vi "SEK2020v1SubVIAlinhar.vi"(9 "Min EV3 Cor":sgl, 10 "Max EV3 Cor":sgl, 11 "NXT/EV3":T1) -> (3 "NXT/EV3 2":T1)   [LabVIEW 2016]
uses:
  <vilib>/NXT/Subs/LVHSConnector.ctl
  <vilib>/NXT/LegoClasses/BrickReference/BrickReference.lvclass
  <vilib>/NXT/Block Support/NXT_OutputPort.ctl
  <vilib>/NXT/Block Support/NXT_InputPort.ctl
  <vilib>/NXT/Dual Mode Library/Sensors/EV3_Color_Reflect.vi
  <vilib>/NXT/NXTIO Xnodes/NXTIONodeSubVIs/NXTMoveMotors.vi
  <vilib>/NXT/NXTIO Xnodes/NXTIONodeSubVIs/NXTStopMotors.vi
  <vilib>/NXT/NXTIO Xnodes/AddressXNode/NXTIOAddress.xnode
  <vilib>/NXT/NXTIO Xnodes/NXTIOXNode/NXTIO.xnode
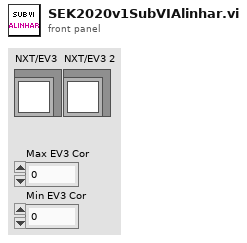
[diagram p1: front panel]
types:
  T1 = typedef "LVHSConnector.ctl" = refnum<class "BrickReference.lvclass">
  T2 = typedef "NXT_InputPort.ctl" = u32
  T3 = typedef "NXT_OutputPort.ctl" = u8
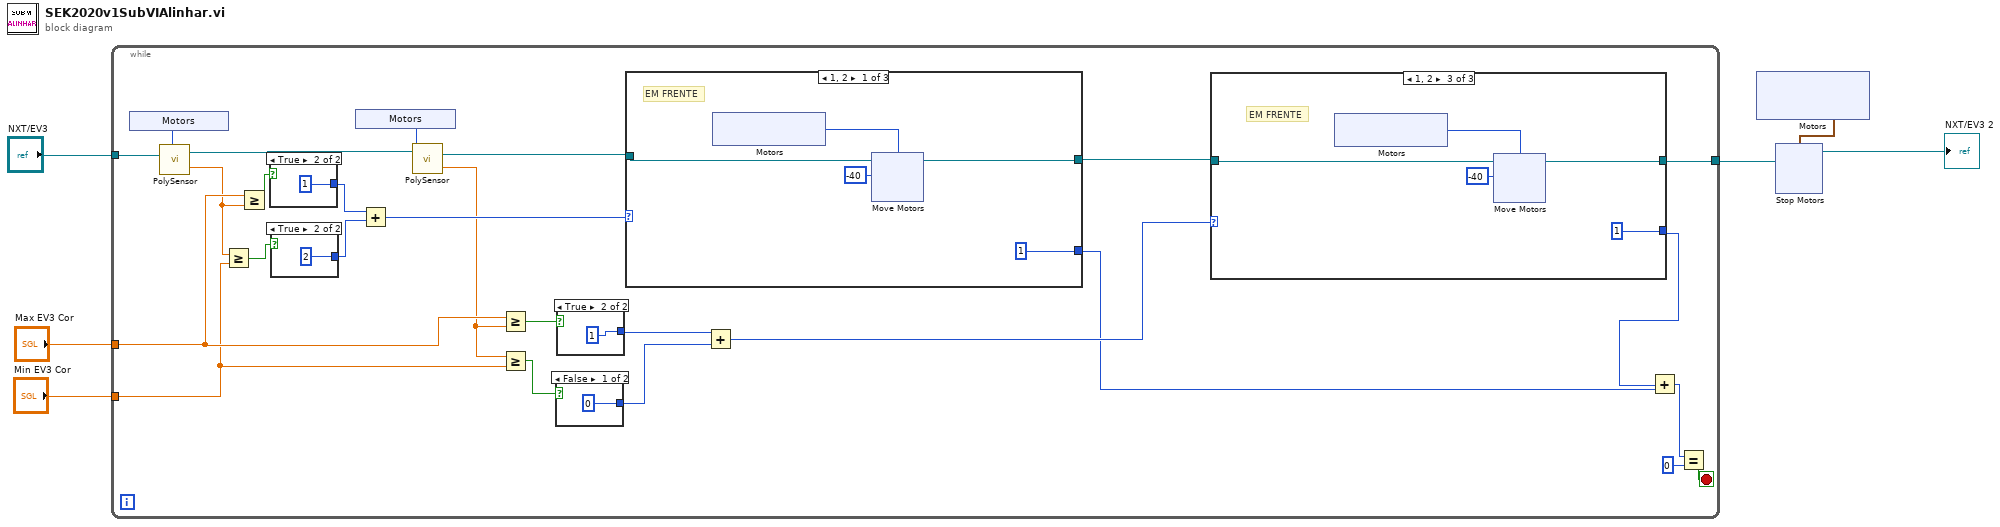
[diagram p0: block diagram]
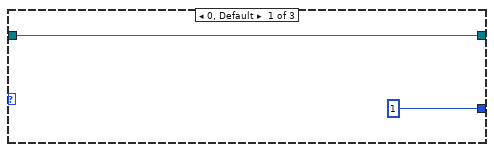
[diagram p2: hidden frame]
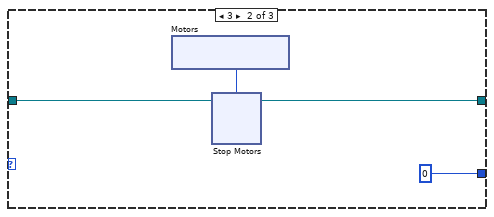
[diagram p3: hidden frame]
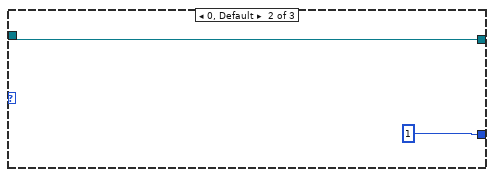
[diagram p4: hidden frame]
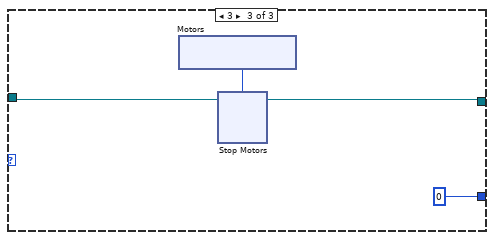
[diagram p5: hidden frame]
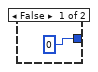
[diagram p6: hidden frame]
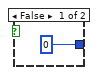
[diagram p7: hidden frame]
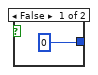
[diagram p8: hidden frame]
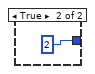
[diagram p9: hidden frame]
diagram:
  n1 = while {
    tunnel: "Max EV3 Cor" -> [w32]
    tunnel: "Min EV3 Cor" -> [w31]
    tunnel: [w11] -> w6
    tunnel: "NXT/EV3" -> [w7]
    stop <- w25 stop-if-true
    n2 = xnode "Motors"() -> ("Sensor"=w13:T2)
    n3 = call-poly <vilib>:"PolySensor.vi"("NXT/EV3"=w7, "Port (Port 1)"=w13) -> ("Scaled Value"=w19:sgl, "NXT/EV3"=w20:T1)  [unwired: 1 in]
    n4 = Greater Or Equal?(x=w19, y=w31) -> (x >= y?=w23:bool)
    n5 = Greater Or Equal?(x=w32, y=w19) -> (x >= y?=w24:bool)
    n6 = case shown="True" w24 {
      tunnel: [0 1] -> w30
      frame False {
      }
      frame True {
      }
    }
    n7 = case shown="True" w23 {
      tunnel: [0 2] -> w29
      frame False {
      }
      frame True {
      }
    }
    n8 = xnode "Motors"() -> ("Sensor"=w12:T2)
    n9 = Add(x=w30, y=w29) -> (x+y=w26:i32)
    n10 = call-poly <vilib>:"PolySensor.vi"("NXT/EV3"=w20, "Port (Port 1)"=w12) -> ("Scaled Value"=w18:sgl, "NXT/EV3"=w17:T1)  [unwired: 1 in]
    n11 = Greater Or Equal?(x=w32, y=w18) -> (x >= y?=w22:bool)
    n12 = Greater Or Equal?(x=w18, y=w31) -> (x >= y?=w21:bool)
    n13 = case shown="False" w21 {
      tunnel: [0 2] -> w27
      frame False {
      }
      frame True {
      }
    }
    n14 = case shown="True" w22 {
      tunnel: [0 1] -> w28
      frame False {
      }
      frame True {
      }
    }
    n15 = case shown="1, 2" w26 {
      tunnel: [w61 w74 w76] -> w15
      tunnel: w17 -> [w62 w74 w77]
      tunnel: [i8 1 ("Power/Speed 1") 1 i8 0 ("Power/Speed 1")] -> w9
      frame 1, 2 {
        # "EM FRENTE"
        n16 = xnode "Motors"() -> ("Motor"=w64:T3)
        n17 = xnode "Move Motors"("Power/Speed 1"=i8 -40, "Motors"=w64, "NXT/EV3"=w62) -> ("NXT/EV3"=w61:T1)
      }
      frame 0, Default {
      }
      frame 3 {
        n18 = xnode "Motors"() -> ("Motor"=w75:T3)
        n19 = xnode "Stop Motors"("Motors"=w75, "NXT/EV3"=w77) -> ("NXT/EV3"=w76:T1)
      }
    }
    n20 = Add(x=w28, y=w27) -> (x+y=w14:i32)
    n21 = case shown="1, 2" w14 {
      tunnel: w15 -> [w36 w38 w49]
      tunnel: [w36 w37 w48] -> w11
      tunnel: [1 i8 0 ("Power/Speed 1") 1] -> w8
      frame 0, Default {
      }
      frame 3 {
        n22 = xnode "Motors"() -> ("Motor"=w39:T3)
        n23 = xnode "Stop Motors"("Motors"=w39, "NXT/EV3"=w38) -> ("NXT/EV3"=w37:T1)
      }
      frame 1, 2 {
        # "EM FRENTE"
        n24 = xnode "Motors"() -> ("Motor"=w50:T3)
        n25 = xnode "Move Motors"("Power/Speed 1"=i8 -40, "Motors"=w50, "NXT/EV3"=w49) -> ("NXT/EV3"=w48:T1)
      }
    }
    n26 = Add(x=w8, y=w9) -> (x+y=w10:i32)
    n27 = Equal?(x=w10, y=i8 0 ("Power/Speed 1")) -> (x = y?=w25:bool)
  }
  n28 = xnode "Motors"() -> ("Motor"=w5:cluster{"Port":T3, "Port":T3})
  n29 = xnode "Stop Motors"("Motors"=w5, "NXT/EV3"=w6) -> ("NXT/EV3"=→"NXT/EV3 2":T1)
